vi "Stereo - Compute Camera Model.vi"(10 "Images and Reference Points in":T4(array[cluster]), 11 "Images":T1[](array[typedef])) -> (1 "Boolean":bool, 2 "Images and Reference Points out":T4(array[cluster]), 3 "Calibrated Images":T1[](array[typedef]))   [LabVIEW 2014]
doc: "Computes a grid coverage based on the Grid Images input array. The result is stored in the image provided as an input."
uses:
  <vilib>/vision/Image Controls.llb/IMAQ Image.ctl
  <vilib>/vision/Calibration.llb/Calibration Reference Points.ctl
  Stereo - Global Variables.vi
panel:
  # "Overview: Computes the camera model calibration for the left and right images."
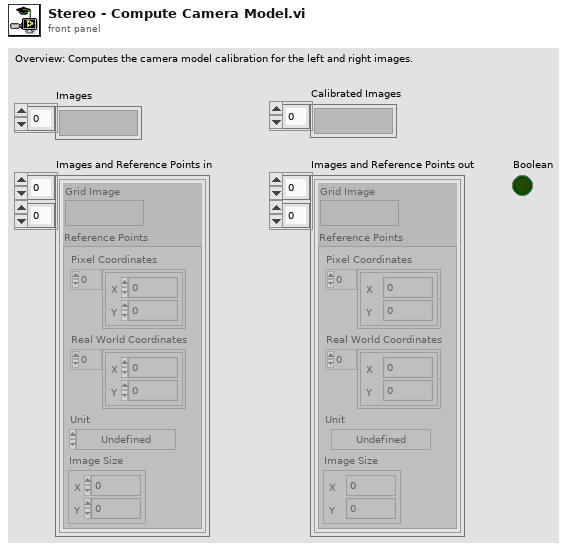
[diagram p1: front panel]
types:
  T1 = typedef "IMAQ Image.ctl" = refnum<image>
  T2 = typedef "Calibration Reference Points.ctl" = cluster{"Pixel Coordinates":cluster{"X":dbl, "Y":dbl}[], "Real World Coordinates":cluster{"X":dbl, "Y":dbl}[], "Unit":T3, "Image Size":cluster{"X":u32, "Y":u32}}
  T3 = typedef "Image Unit" = enum32{"Undefined", "Angström", "Micrometer", "Millimeter", "Centimeter", "Meter", "Kilometer", "Microinch", "Inch", "Feet", "Nautical miles", "Standard miles", "Steps"}
  T4 = cluster{"Grid Image":T1, "Reference Points":T2}[][]
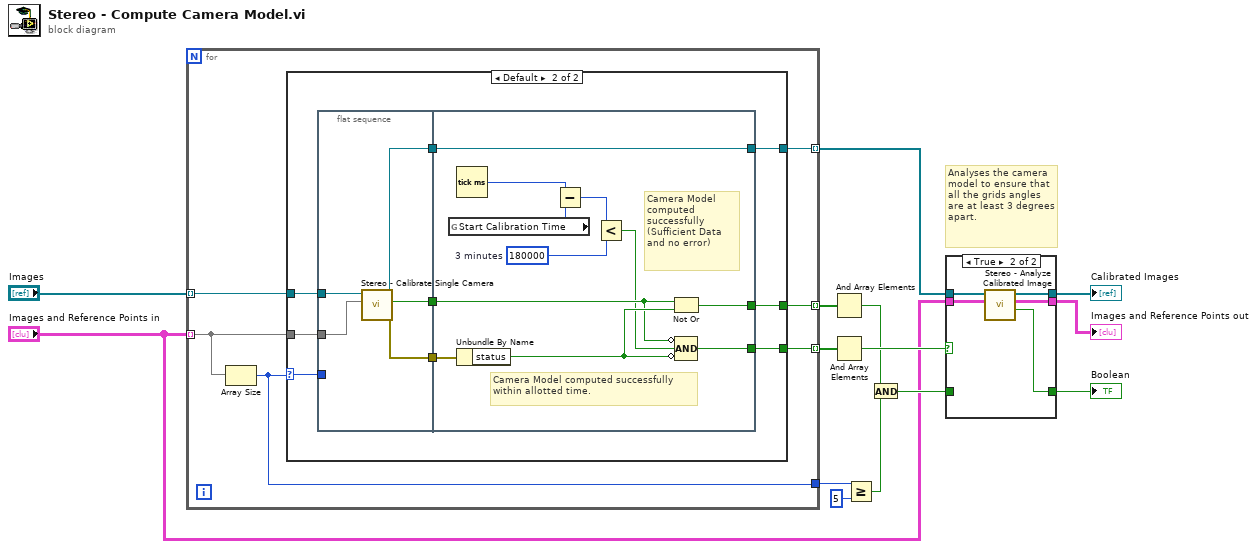
[diagram p0: block diagram]
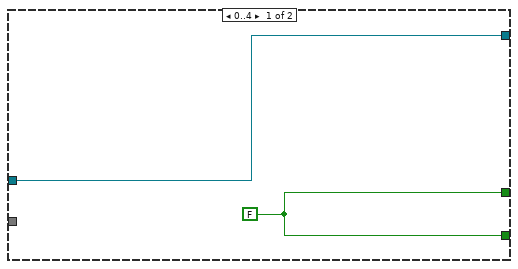
[diagram p2: hidden frame]
diagram:
  # "Analyses the camera model to ensure that all the grids angles are at least 3 degrees apart."
  n1 = for {
    tunnel: "Images and Reference Points in" -> [w20] mode=indexing
    tunnel: "Images" -> [w19] mode=indexing
    tunnel: [w18] -> w12 mode=indexing
    tunnel: [w17] -> w11 mode=indexing
    tunnel: [w16] -> w7
    tunnel: [w15] -> w6 mode=indexing
    n2 = Array Size(array=w20) -> (size(s)=w16:i32)
    n3 = case shown="Default" w16 {
      selector: w16 -> [_ w31]
      tunnel: w20 -> [_ w29]
      tunnel: w19 -> [w21 w30]
      tunnel: [w22 w27] -> w18
      tunnel: [w22 w26] -> w17
      tunnel: [w21 w24] -> w15
      frame 0..4 {
        w22 = FALSE
      }
      frame Default {
        n4 = flat-sequence {
          tunnel: w31 -> [_]
          tunnel: w29 -> [w33]
          tunnel: w30 -> [w34]
          tunnel: [w35] -> w28
          tunnel: [w36] -> w25
          tunnel: [w32] -> w23
          tunnel: w28 -> [w42]
          tunnel: [w43] -> w27
          tunnel: [w41] -> w26
          tunnel: w25 -> [w39]
          tunnel: [w37] -> w24
          tunnel: w23 -> [w37]
          frame #0 {
            n5 = call "Stereo - Calibrate Single Camera.vi"("Calibration Grids"=w33, "Image in"=w34) -> ("error out"=w35:errorcluster, "Insufficient Data"=w36:bool, "Image out"=w32:T1)  [unwired: 1 in, 6 out]
          }
          frame #1 {
            w45 = u32 180000  # 3 minutes
            # "Camera Model computed successfully (Sufficient Data and no error)"
            # "Camera Model computed successfully within allotted time."
            n6 = global read "Stereo - Global Variables.vi" "Start Calibration Time"() -> (w47:u32)
            n7 = Tick Count (ms)() -> (millisecond timer value=w44:u32)
            n8 = Unbundle By Name(w42) -> ("status"=w40:bool)
            n9 = Subtract(x=w44, y=w47) -> (x-y=w46:u32)
            n10 = Less?(x=w46, y=w45) -> (x < y?=w38:bool)
            n11 = Not Or(1:w40, 2:w39) -> (0:w41:bool)
            n12 = Compound Arithmetic op=AND(invert w39, w38, invert w40) -> (w43:bool)
          }
        }
      }
    }
  }
  n13 = And Array Elements(Boolean array=w11) -> (logical AND=w10:bool)
  n14 = And Array Elements(Boolean array=w12) -> (logical AND=w14:bool)
  n15 = Greater Or Equal?(x=w7, y=5) -> (x >= y?=w9:bool)
  n16 = And(x=w10, y=w9) -> (x .and. y?=w13:bool)
  n17 = case shown="True" w14 {
    tunnel: [w50 w55] -> w5
    tunnel: w6 -> [w50 w54]
    tunnel: [w48 w52] -> w1
    tunnel: [w49 w53] -> w3
    tunnel: "Images and Reference Points in" -> [w49 w51]
    tunnel: w13 -> [w48 _]
    frame False {
    }
    frame True {
      n18 = call "Stereo - Analyze Calibrated Image.vi"("Grid Images in"=w51, "Calibrated Images in"=w54) -> ("Calibration OK"=w52:bool, "Grid Images out"=w53:T4, "Calibrated Images out"=w55:T1[])  [unwired: 1 in, 6 out]
    }
  }
  "Calibrated Images" <- w5
  "Images and Reference Points out" <- w3
  "Boolean" <- w1
